vi "GaussRakeSimulator.vi"() -> ()   [LabVIEW 2011]
panel:
  in  "JitterFraction":dbl=0.2
  in  "Mode":string(combo)="WhatToDo"
  in  "Rake Points (n)":u32=3
  out "Xdata":dbl[](array[numeric])
  out "Ydata":dbl[](array[numeric])
  in  "Rake Spacing":dbl=55.0
  in  "Rake Centre Position":dbl
  in  "Spread":dbl
  in  "Center":dbl
  in  "Amplitude":dbl
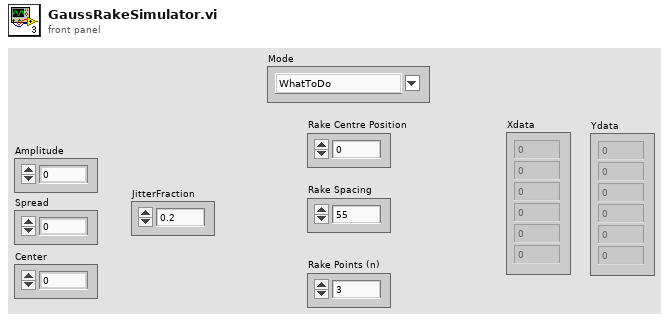
[diagram p1: front panel]
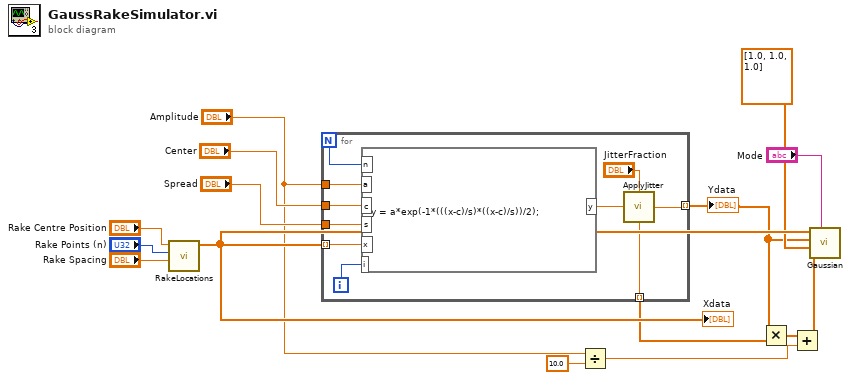
[diagram p0: block diagram]
diagram:
  n1 = call "RakeLocations.vi"("Rake Spacing"="Rake Spacing", "Rake Points (n)"="Rake Points (n)", "Rake Centre Position"="Rake Centre Position") -> ("Locations"=w10:dbl[])  [unwired: 8 in]
  "Xdata" <- w10
  n2 = for {
    N -> [w20]
    tunnel: "Amplitude" -> [w24]
    tunnel: "Center" -> [w22]
    tunnel: "Spread" -> [w23]
    tunnel: [w17] -> w7 mode=indexing
    tunnel: w10 -> [w21] mode=indexing
    tunnel: ["JitterFraction"] -> w6 mode=indexing
    i -> [w19]
    n3 = formula code="y = a*exp(-1*(((x-c)/s)*((x-c)/s))/2);"("a"=w24, "c"=w22, "s"=w23, "i"=w19, "x"=w21, "n"=w20) -> ("y"=w18:dbl)
    n4 = call "ApplyJitter.vi"("ValueIn"=w18, "JitterFraction"="JitterFraction") -> ("JitteredValueOut"=w17:dbl)
  }
  "Ydata" <- w7
  n5 = Divide(x="Amplitude", y=10.0) -> (x/y=w1:dbl)
  n6 = Multiply(x=w7, y=w6) -> (x*y=w2:dbl[])
  n7 = Add(x=w2, y=w1) -> (x+y=w5:dbl[])
  n8 = call "Gaussian.vi"("Mode"="Mode", "YerrorIn"=w5, "XerrorIn"=dbl[] [1.0, 1.0, 1.0], "YdataIn"=w7, "XdataIn"=w10) -> ()  [unwired: 2 in, 5 out]
